vi "Overlay result.vi"(8 "error in (no error)":errorcluster, 9 "Size":i32=20, 10 "Array":dbl[](array[numeric]), 11 "Image in":T1) -> (0 "error out":errorcluster, 3 "Image out":T1)   [LabVIEW 2018]
uses:
  <vilib>/vision/Image Controls.llb/IMAQ Image.ctl
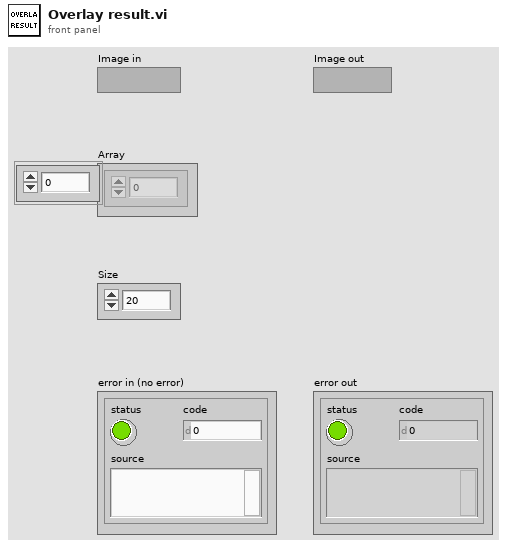
[diagram p1: front panel]
types:
  T1 = typedef "IMAQ Image.ctl" = refnum<image>
  T2 = cluster{"Desired Font (Application)":enum16{"User-specified Font", "Application Font", "System Font", "Dialog Font"}, "[User-specified Font]":cluster{"Font Name":string, "Size":i16, "Strikeout?":bool, "Italic?":bool, "Underline?":bool, "Outline?":bool, "Shadow?":bool, "Bold?":bool, "Rotation Angle":dbl}, "Horizontal Alignment":i16, "Vertical Alignment":i16}
  T3 = cluster{"Left":i32, "Top":i32, "Right":i32, "Bottom":i32}
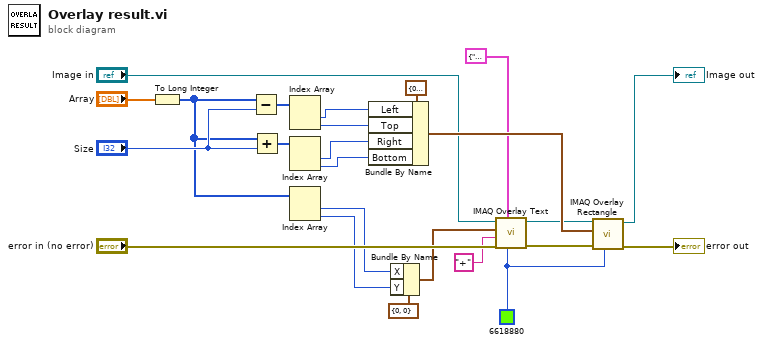
[diagram p0: block diagram]
diagram:
  w10 = u32 6618880 ("Color")
  n1 = To Long Integer(number="Array") -> (32bit integer=w3:i32[])
  n2 = Subtract(x=w3, y="Size") -> (x-y=w17:i32[])
  n3 = Add(x=w3, y="Size") -> (x+y=w19:i32[])
  n4 = Index Array(array=w17) -> (element #1=w8:i32, element #2=w7:i32)  [unwired: 2 in]
  n5 = Index Array(array=w19) -> (element #1=w20:i32, element #2=w21:i32)  [unwired: 2 in]
  n6 = Index Array(array=w3) -> (element #1=w2:i32, element #2=w1:i32)  [unwired: 2 in]
  n7 = Bundle By Name(cluster=T3 {"Left"=0, "Top"=0, "Right"=0, "Bottom"=0} ("Rectangle"), "Left"=w8, "Top"=w7, "Right"=w20, "Bottom"=w21) -> (w22:T3)
  n8 = Bundle By Name(cluster=cluster{"X":i32, "Y":i32} {"X"=0, "Y"=0} ("Origin"), "X"=w2, "Y"=w1) -> (w6:cluster{"X":i32, "Y":i32})
  n9 = call "IMAQ Overlay Text"("Text Color (black)"=w10, "Font, Size & Style"=T2 {"Desired Font (Application)"=enum."Application Font", "[User-specified Font]"={"Font Name"="", "Size"=20, "Strikeout?"=FALSE, "Italic?"=FALSE, "Underline?"=FALSE, "Outline?"=FALSE, "Shadow?"=FALSE, "Bold?"=FALSE, "Rotation Angle"=0.0}, "Horizontal Alignment"=1, "Vertical Alignment"=2}, "error in (no error)"="error in (no error)", "String"="+", "Origin"=w6, "Image"="Image in") -> ("error out"=w13:errorcluster, "Image Out"=w11:T1)  [unwired: 4 in]
  n10 = call "IMAQ Overlay Rectangle"("Color"=w10, "error in (no error)"=w13, "Rectangle"=w22, "Image"=w11) -> ("error out"=→"error out":errorcluster, "Image Out"=→"Image out":T1)  [unwired: 6 in]
